vi "Position Control.vi"(10 "FMS Desired Color":string, 11 "Color Sensor Input":string) -> (3 "Are we done?":bool)   [LabVIEW 2019]
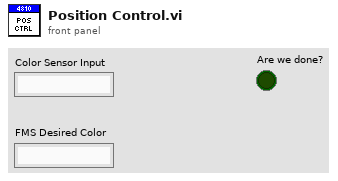
[diagram p1: front panel]
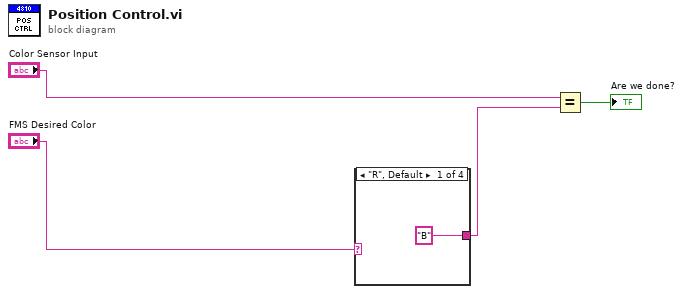
[diagram p0: block diagram]
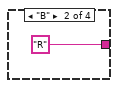
[diagram p2: hidden frame]
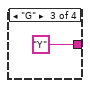
[diagram p3: hidden frame]
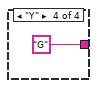
[diagram p4: hidden frame]
diagram:
  n1 = case shown="\"R\", Default" "FMS Desired Color" {
    tunnel: ["B" "R" "Y" "G"] -> w1
    frame "R", Default {
    }
    frame "B" {
    }
    frame "G" {
    }
    frame "Y" {
    }
  }
  n2 = Equal?(x="Color Sensor Input", y=w1) -> (x = y?=→"Are we done?":bool)
